vi "pcb_select_pixel_tcp.vi"(8 "error in (no error)":errorcluster, 9 "Cell":u32, 10 "Pixel":u32) -> (0 "error out":errorcluster, 2 "Pixel set?":bool)   [LabVIEW 2018]
panel:
  out "IP address out":string="192.168.137.152"
  out "disconnect msg":string
  out "disconnect bytes written":i32
  out "select pixel bytes written":i32
  out "select pixel msg":string
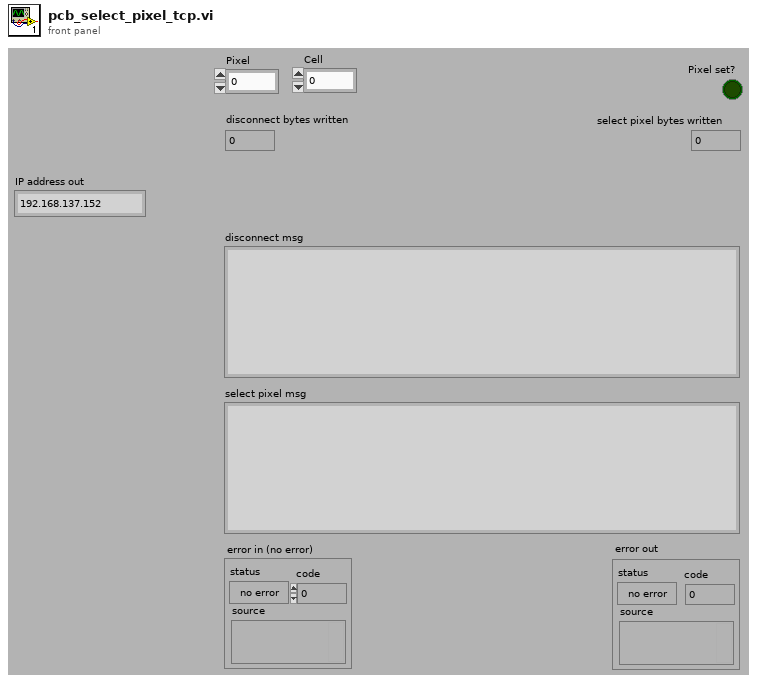
[diagram p1: front panel]
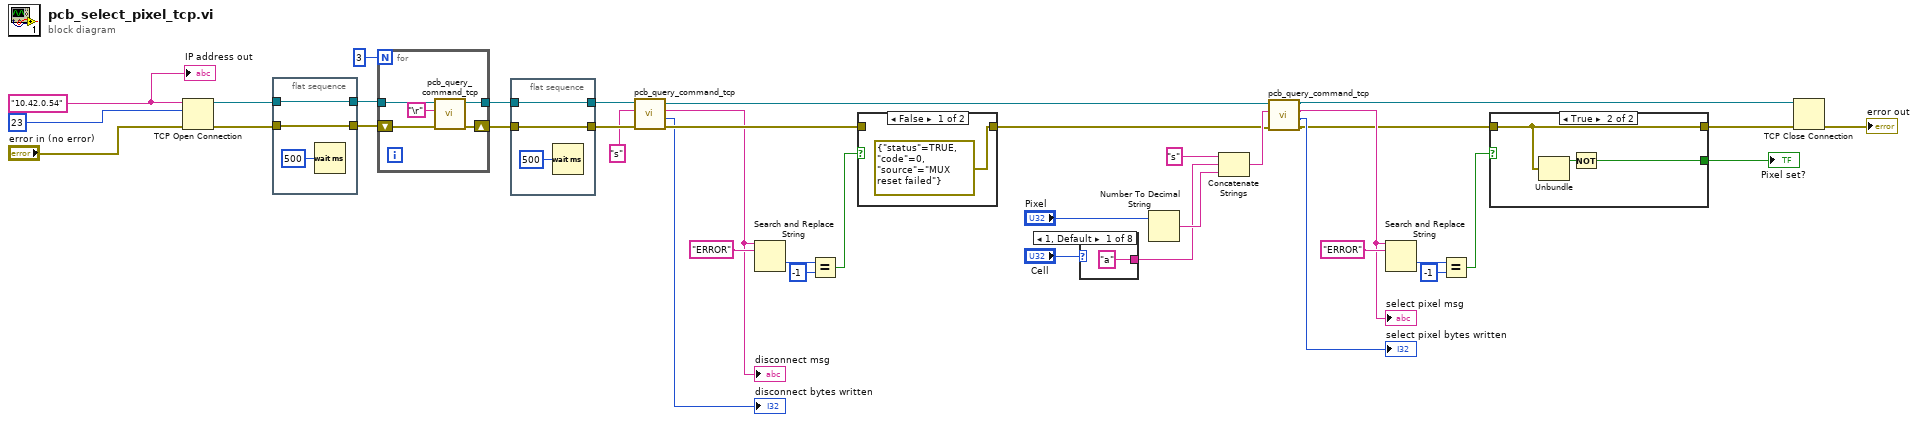
[diagram p0: block diagram]
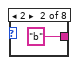
[diagram p2: hidden frame]
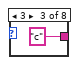
[diagram p3: hidden frame]
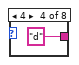
[diagram p4: hidden frame]
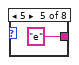
[diagram p5: hidden frame]
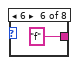
[diagram p6: hidden frame]
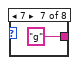
[diagram p7: hidden frame]
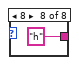
[diagram p8: hidden frame]
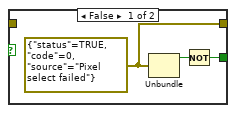
[diagram p9: hidden frame]
diagram:
  w25 = "10.42.0.54" ("IP address")
  n1 = TCP Open Connection(address=w25, remote port or service name=u16 23, error in (no error)="error in (no error)") -> (connection ID=w20:refnum<k5>, error out=w19:errorcluster)  [unwired: 2 in]
  n2 = flat-sequence {
    tunnel: [w42] -> w18
    tunnel: w20 -> [w42]
    tunnel: [w41] -> w17
    tunnel: w19 -> [w41]
    frame #0 {
      n3 = Wait (ms)(milliseconds to wait=u32 500) -> ()  [unwired: 1 out]
    }
  }
  n4 = for {
    N: 3 -> [_]
    shift-right: [w47] -> w21
    shift-left: w17 -> [w44]
    tunnel: w18 -> [w45]
    tunnel: [w46] -> w22
    n5 = call "pcb_query_command_tcp.vi"("error in (no error)"=w44, "command"="\r", "connection ID"=w45) -> ("error out"=w47:errorcluster, "connection ID out"=w46:refnum<k5>)  [unwired: 5 in, 2 out]
  }
  n6 = flat-sequence {
    tunnel: [w50] -> w13
    tunnel: w22 -> [w50]
    tunnel: [w49] -> w12
    tunnel: w21 -> [w49]
    frame #0 {
      n7 = Wait (ms)(milliseconds to wait=u32 500) -> ()  [unwired: 1 out]
    }
  }
  n8 = call "pcb_query_command_tcp.vi"("error in (no error)"=w12, "command"="s" ("string"), "connection ID"=w13) -> ("error out"=w10:errorcluster, "bytes written"=→"disconnect bytes written":i32, "output"=w9:string, "connection ID out"=w1:refnum<k5>)  [unwired: 5 in]
  "disconnect msg" <- w9
  n9 = Search and Replace String(input string=w9, search string="ERROR") -> (offset past replacement=w38:i32)  [unwired: 6 in, 3 out]
  n10 = Equal?(x=w38, y=-1) -> (x = y?=w36:bool)
  n11 = case shown="False" w36 {
    tunnel: w10 -> [_ w52]
    tunnel: [errorcluster {"status"=TRUE, "code"=0, "source"="MUX reset failed"} ("error in (no error) 2") w52] -> w6
    frame False {
    }
    frame True {
    }
  }
  n12 = case shown="1, Default" "Cell" {
    tunnel: ["a" ("string") "b" ("string") "c" ("string") "d" ("string") "e" ("string") "f" ("string") "g" ("string") "h" ("string")] -> w26
    frame 1, Default {
    }
    frame 2 {
    }
    frame 3 {
    }
    frame 4 {
    }
    frame 5 {
    }
    frame 6 {
    }
    frame 7 {
    }
    frame 8 {
    }
  }
  n13 = Number To Decimal String(number="Pixel") -> (decimal integer string=w29:string)  [unwired: 1 in]
  n14 = Concatenate Strings("s" ("string"), w26, w29) -> (w7:string)
  n15 = call "pcb_query_command_tcp.vi"("error in (no error)"=w6, "command"=w7, "connection ID"=w1) -> ("error out"=w2:errorcluster, "bytes written"=→"select pixel bytes written":i32, "output"=w4:string, "connection ID out"=w5:refnum<k5>)  [unwired: 5 in]
  "select pixel msg" <- w4
  n16 = Search and Replace String(input string=w4, search string="ERROR") -> (offset past replacement=w32:i32)  [unwired: 6 in, 3 out]
  n17 = Equal?(x=w32, y=-1) -> (x = y?=w30:bool)
  n18 = case shown="True" w30 {
    tunnel: [w63 w64] -> w15
    tunnel: [w61 w66] -> w35
    tunnel: w2 -> [_ w64]
    frame False {
      w63 = errorcluster {"status"=TRUE, "code"=0, "source"="Pixel select failed"} ("error in (no error) 2")
      n19 = Unbundle(w63) -> ("status"=w62:bool)  [unwired: 2 out]
      n20 = Not(x=w62) -> (.not. x?=w61:bool)
    }
    frame True {
      n21 = Unbundle(w64) -> ("status"=w65:bool)  [unwired: 2 out]
      n22 = Not(x=w65) -> (.not. x?=w66:bool)
    }
  }
  "Pixel set?" <- w35
  n23 = TCP Close Connection(connection ID=w5, error in (no error)=w15) -> (error out=→"error out":errorcluster)  [unwired: 1 in, 1 out]
  "IP address out" <- w25
